vi "GetDstMatSize.vi"(9 "dSize":T2, 10 "SrcHeight":i32, 11 "SrcWidth":i32) -> (3 "Size":T1)   [LabVIEW 2020, in "OpenLvVision_OpenCv.lvlib"]
uses:
  OpenLvVision_OpenCv.lvlib
  TypeDef/Point/2D_PointI32.ctl
  TypeDef/Size.ctl
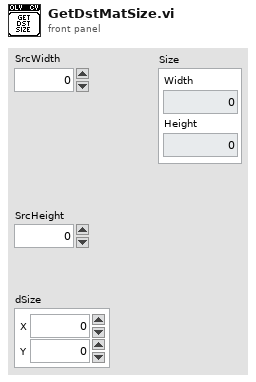
[diagram p1: front panel]
types:
  T1 = typedef "OpenLvVision_OpenCv.lvlib/Size.ctl" = cluster{"Width":i32, "Height":i32}
  T2 = typedef "OpenLvVision_OpenCv.lvlib/2D_PointI32.ctl" = cluster{"X":i32, "Y":i32}
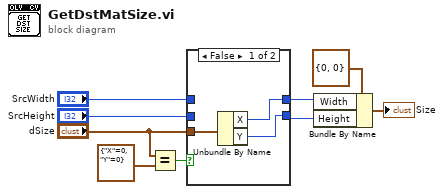
[diagram p0: block diagram]
diagram:
  n1 = Equal?(x="dSize", y=T2 {"X"=0, "Y"=0} ("Point")) -> (x = y?=w9:bool)
  n2 = case shown="False" w9 {
    tunnel: [w11 w13] -> w4
    tunnel: [w10 w14] -> w3
    tunnel: "dSize" -> [w12 _]
    tunnel: "SrcHeight" -> [_ w14]
    tunnel: "SrcWidth" -> [_ w13]
    frame False {
      n3 = Unbundle By Name(w12) -> ("X"=w11:i32, "Y"=w10:i32)
    }
    frame True {
    }
  }
  n4 = Bundle By Name(cluster=T1 {"Width"=0, "Height"=0} ("Size"), "Width"=w4, "Height"=w3) -> (→"Size":T1)
